vi "test.vi"() -> ()   [LabVIEW 2018]
panel:
  out "2":i32
  out "3":i32
  in  "stop":bool
  out "1":i32
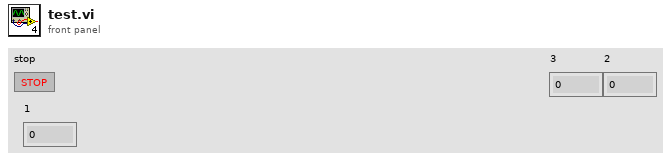
[diagram p1: front panel]
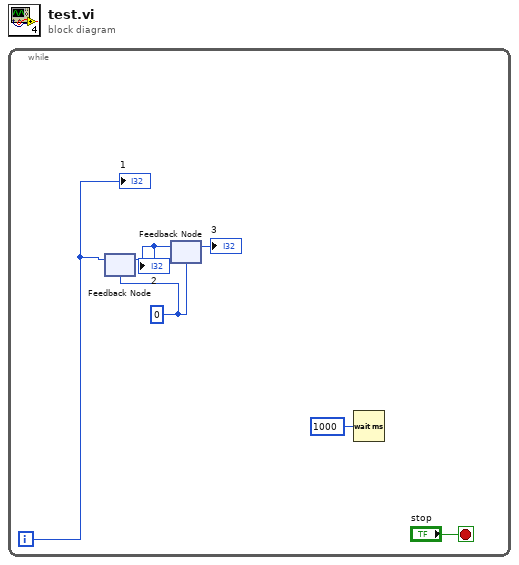
[diagram p0: block diagram]
diagram:
  n1 = while {
    i -> [w4]
    stop <- "stop" stop-if-true
    w2 = 0
    n2 = feedback-in #1(w4) -> ()
    n3 = feedback #1(w2) -> (w3:i32)
    "2" <- w3
    n4 = feedback #2(w2) -> (→"3":i32)
    n5 = feedback-in #2(w3) -> ()
    n6 = Wait (ms)(milliseconds to wait=u32 1000) -> ()  [unwired: 1 out]
    "1" <- w4
  }
